vi "Configure Client.vi"(8 "error in (no error)":errorcluster, 10 "Client in":refnum<class "Connection.lvclass">, 11 "TcpResource in":refnum<class "TcpResource.lvclass">) -> (0 "error out":errorcluster, 2 "Client":refnum<class "Connection.lvclass">, 3 "TcpResource out":refnum<class "TcpResource.lvclass">)   [LabVIEW 2020, in "PicoG-Core.lvlib" / "TcpResource.lvclass"]
uses:
  TcpResource.lvclass
  TcpResource.lvclass/TcpResource.ctl
  <vilib>/IlluminatedG/lv-stream-tcp/Stream-TCP.lvlib
  <vilib>/IlluminatedG/lv-stream/Endpoint/Endpoint.lvclass
  <vilib>/IlluminatedG/lv-stream/Connection/Connection.lvclass
  C:/Program Files (x86)/National Instruments/LabVIEW 2020/vi.lib/IlluminatedG/lv-stream/Endpoint/Endpoint.lvclass
  C:/Program Files (x86)/National Instruments/LabVIEW 2020/vi.lib/IlluminatedG/lv-stream/Connection/Connection.lvclass
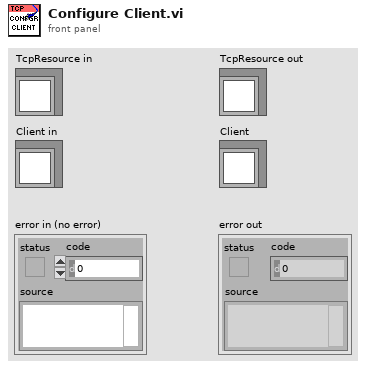
[diagram p1: front panel]
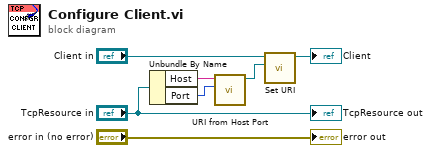
[diagram p0: block diagram]
diagram:
  n1 = Unbundle By Name("TcpResource in") -> ("Host"=w5:string, "Port"=w4:u16)
  n2 = call <vilib>:"URI from Host Port.vi"("Port"=w4, "Host"=w5) -> ("URI"=w2:refnum<class "URI.lvclass">)  [unwired: 9 in]
  n3 = call <vilib>:"Set URI.vi"("URI"=w2, "Endpoint in"="Client in") -> ("Endpoint out"=→"Client":refnum<class "Connection.lvclass">)  [unwired: 8 in, 1 out]
  "error out" <- "error in (no error)"
  "TcpResource out" <- "TcpResource in"
